vi "Open.vi"(6 "Start Counter":bool=TRUE, 7 "Allow multiple opens?":bool, 8 "error in (no error)":errorcluster, 9 "Encoder Signal Mode":T1, 10 "Channel Name":tag) -> (0 "error out":errorcluster, 3 "Encoder Ref Out":T2)   [LabVIEW 2021, in "Encoder.lvlib"]
doc: "Opens a reference to an encoder channel. You must open a reference before you use an encoder channel to read and decode signals from an encoder."
uses:
  <vilib>/myRIO/Instrument Drivers/Onboard IO/Encoder/Encoder.lvlib
  <vilib>/myRIO/Instrument Drivers/Onboard IO/Encoder/typedefs/Encoder Reference.ctl
  <vilib>/myRIO/Common/Instrument Driver Framework/Utilities/typedefs/myRIO Generic Hardware Reference.ctl
  <vilib>/myRIO/Common/Instrument Driver Framework/Utilities/typedefs/Hardware Version Enum.ctl
  <vilib>/myRIO/Common/Instrument Driver Framework/Utilities/typedefs/myRIO v1.0 Reference.ctl
  <vilib>/myRIO/Common/Instrument Driver Framework/Utilities/typedefs/Generic FPGA Reference.ctl
  <vilib>/myRIO/Common/Instrument Driver Framework/myRIO v1.0/Encoder/typedefs/Encoder Channels Enum.ctl
  <vilib>/myRIO/Common/Instrument Driver Framework/myRIO v1.0/Encoder/typedefs/Encoder Signal Mode.ctl
  <vilib>/myRIO/Common/Instrument Driver Framework/myRIO v1.0/Encoder/typedefs/Encoder Configuration v1.0.ctl
  <vilib>/myRIO/Common/Instrument Driver Framework/Utilities/vis/Validate Channels.vi
  <vilib>/myRIO/Common/Instrument Driver Framework/myRIO v1.0/Encoder/vis/myRIO v1.0 Reserve Encoder.vi
  <vilib>/myRIO/Common/Instrument Driver Framework/myRIO v1.0/Encoder/vis/myRIO v1.0 Unreserve Encoder.vi
  <vilib>/myRIO/Common/Instrument Driver Framework/roboRIO v1.0/Encoder/vis/roboRIO v1.0 Reserve Encoder.vi
  <vilib>/myRIO/Common/Instrument Driver Framework/ELVIS III v1.0/Encoder/vis/ELVIS III v1.0 Reserve Encoder.vi
  <vilib>/myRIO/Common/Instrument Driver Framework/myRIO v1.0/Encoder/vis/myRIO v1.0 Build MUX Configuration Encoder.vi
  <vilib>/myRIO/Common/Instrument Driver Framework/myRIO v1.0/Resource Manager/vis/myRIO v1.0 Reserve Channel List.vi
  <vilib>/myRIO/Common/Instrument Driver Framework/myRIO v1.0/Resource Manager/vis/myRIO v1.0 Unreserve Channel List.vi
  <vilib>/myRIO/Common/Instrument Driver Framework/roboRIO v1.0/Encoder/vis/roboRIO v1.0 Build MUX Configuration Encoder.vi
  <vilib>/myRIO/Common/Instrument Driver Framework/roboRIO v1.0/Resource Manager/vis/roboRIO v1.0 Reserve Channel List.vi
  <vilib>/myRIO/Common/Instrument Driver Framework/ELVIS III v1.0/Encoder/vis/ELVIS III v1.0 Build MUX Configuration Encoder.vi
  <vilib>/myRIO/Common/Instrument Driver Framework/myRIO v1.0/Resource Manager/vis/myRIO v1.0 Create Configuration List.vi
  <vilib>/myRIO/Common/Instrument Driver Framework/myRIO v1.0/Resource Manager/vis/myRIO v1.0 Reserve Channel.vi
  <vilib>/myRIO/Common/Instrument Driver Framework/myRIO v1.0/Resource Manager/vis/myRIO v1.0 Unreserve Channel.vi
  <vilib>/myRIO/Common/Instrument Driver Framework/roboRIO v1.0/Resource Manager/vis/roboRIO v1.0 Create Configuration List.vi
  <vilib>/myRIO/Common/Instrument Driver Framework/roboRIO v1.0/Resource Manager/vis/roboRIO v1.0 Reserve Channel.vi
  <vilib>/myRIO/Common/Instrument Driver Framework/roboRIO v1.0/Resource Manager/vis/roboRIO v1.0 Unreserve Channel.vi
  <vilib>/myRIO/Common/Instrument Driver Framework/ELVIS III v1.0/Resource Manager/vis/ELVIS III v1.0 Create Configuration List.vi
  <vilib>/myRIO/Common/Instrument Driver Framework/myRIO v1.0/Resource Manager/vis/myRIO v1.0 Build Mutex Name.vi
  <vilib>/myRIO/Common/Instrument Driver Framework/roboRIO v1.0/Resource Manager/vis/roboRIO v1.0 Build Mutex Name.vi
  <vilib>/Utility/VariantDataType/GetNumericInfo.vi
  <vilib>/myRIO/Common/Instrument Driver Framework/Utilities/vis/IO Manager.vi
  <vilib>/myRIO/Common/Instrument Driver Framework/Utilities/vis/Configuration Manager.vi
  <vilib>/myRIO/Common/Instrument Driver Framework/myRIO v1.0/Resource Manager/vis/myRIO v1.0 Configure IO.vi
  <vilib>/myRIO/Common/Instrument Driver Framework/myRIO v1.0/myRIO v1.0 Close.vi
  <vilib>/myRIO/Common/Instrument Driver Framework/myRIO v1.0/Encoder/vis/myRIO v1.0 Shutdown Encoder.vi
  <vilib>/myRIO/Common/Instrument Driver Framework/roboRIO v1.0/Resource Manager/vis/roboRIO v1.0 Configure IO.vi
  <vilib>/myRIO/Common/Instrument Driver Framework/ELVIS III v1.0/Resource Manager/vis/ELVIS III v1.0 Reserve Channel List.vi
  <vilib>/myRIO/Common/Instrument Driver Framework/ELVIS III v1.0/Resource Manager/vis/ELVIS III v1.0 Configure IO.vi
  <vilib>/userdefined/High Color/nirio_resource_hc.ctl
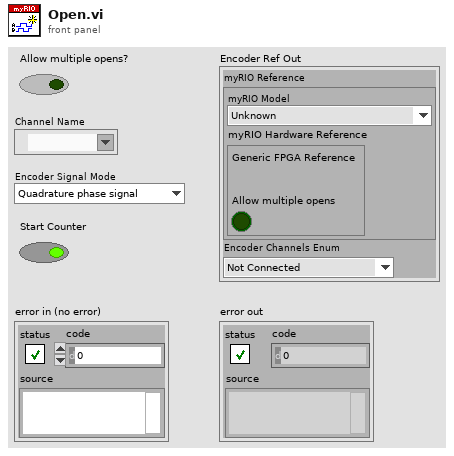
[diagram p1: front panel]
types:
  T1 = typedef "Encoder Signal Mode.ctl" = enum16{"Quadrature phase signal", "Step and direction signal"}
  T2 = typedef "Encoder.lvlib/Encoder Reference.ctl" = cluster{"myRIO Reference":T3, "Encoder Channels Enum":T7}
  T3 = typedef "myRIO Generic Hardware Reference.ctl" = cluster{"myRIO Model":T4, "myRIO Hardware Reference":T5}
  T4 = typedef "Hardware Version Enum.ctl" = enum16{"Unknown", "myRIO-1900", "myRIO-1950", "roboRIO", "NI ELVIS RIO CM", "ELVIS III"}
  T5 = typedef "myRIO v1.0 Reference.ctl" = cluster{"Generic FPGA Reference":T6, "Allow multiple opens":bool}
  T6 = typedef "Generic FPGA Reference.ctl" = refnum<k20>
  T7 = typedef "Encoder Channels Enum.ctl" = enum16{"Not Connected", "C/ENC0", "C/ENC1", "A/ENC", "A/ENC0", "A/ENC1", "A/ENC2", "A/ENC3", "A/ENC4", "A/ENC5", "A/ENC6", "A/ENC7", "A/ENC8", "A/ENC9", "B/ENC", "B/ENC0", "B/ENC1", "B/ENC2", "B/ENC3", "B/ENC4", "B/ENC5", "B/ENC6", "B/ENC7", "B/ENC8", "B/ENC9", "DIO/ENC0", "DIO/ENC1", "DIO/ENC2", "DIO/ENC3", "DIO/ENC4"}
  T8 = typedef "nirio_resource_hc.ctl" = tag
  T9 = typedef "Encoder Configuration v1.0.ctl" = cluster{"Encoder Signal Mode":T1, "Start Counter":bool}
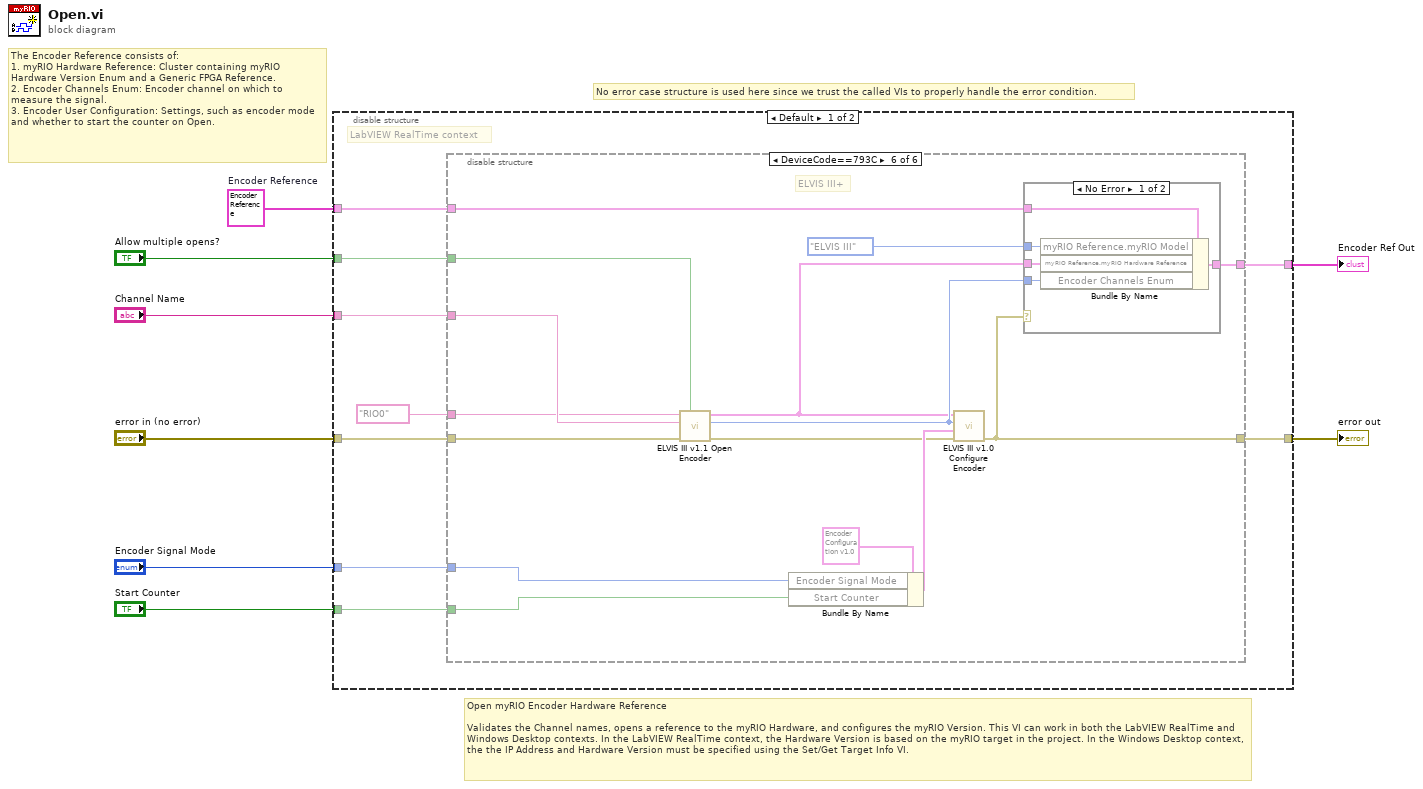
[diagram p0: block diagram]
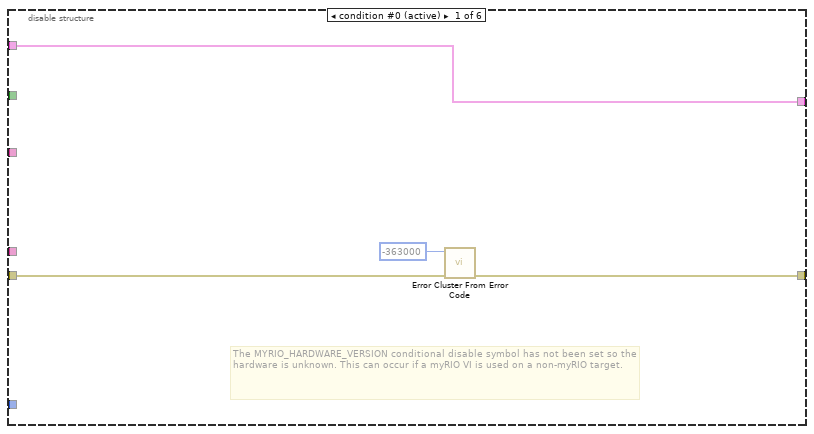
[diagram p2: hidden frame]
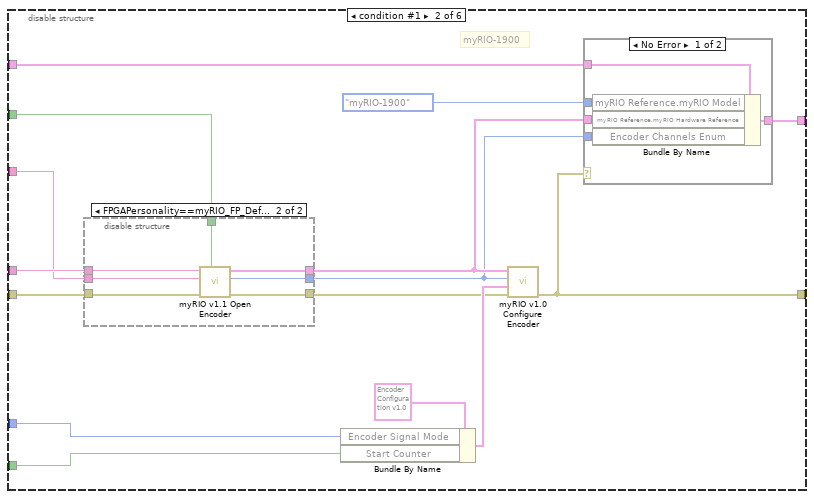
[diagram p3: hidden frame]
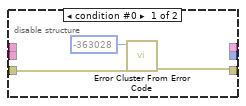
[diagram p4: hidden frame]
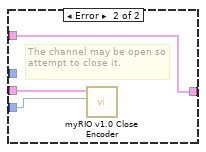
[diagram p5: hidden frame]
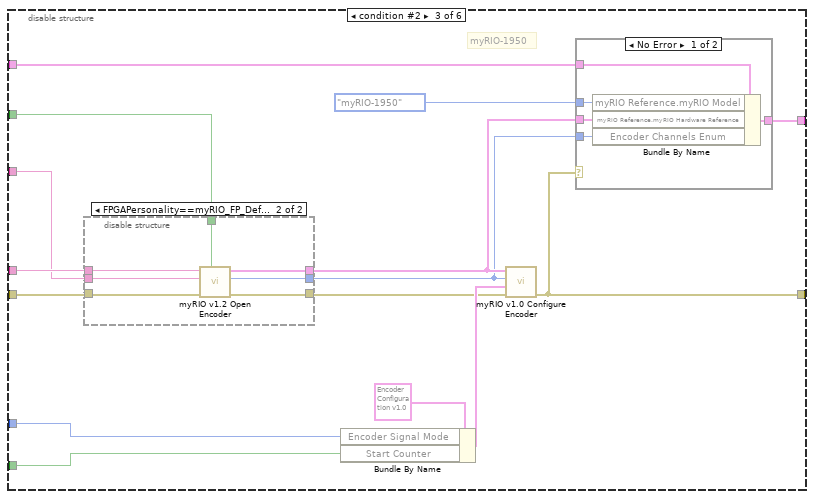
[diagram p6: hidden frame]
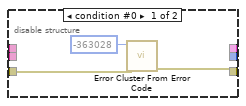
[diagram p7: hidden frame]
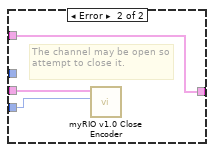
[diagram p8: hidden frame]
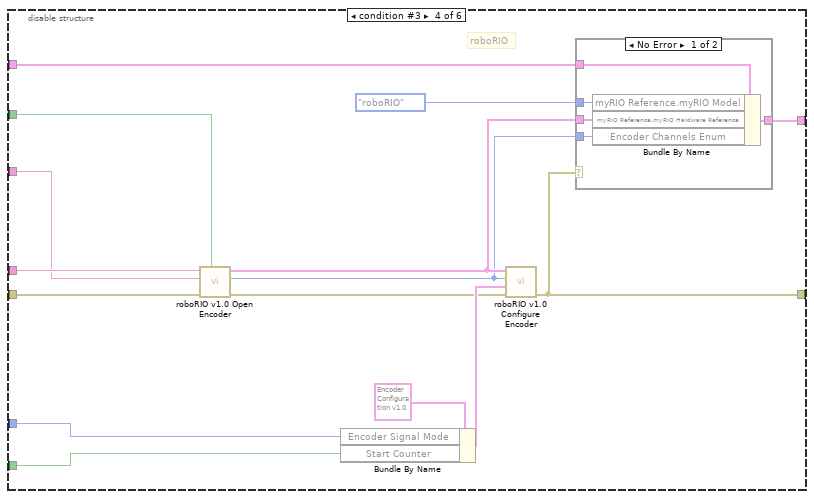
[diagram p9: hidden frame]
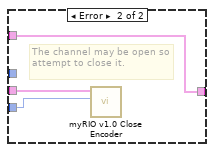
[diagram p10: hidden frame]
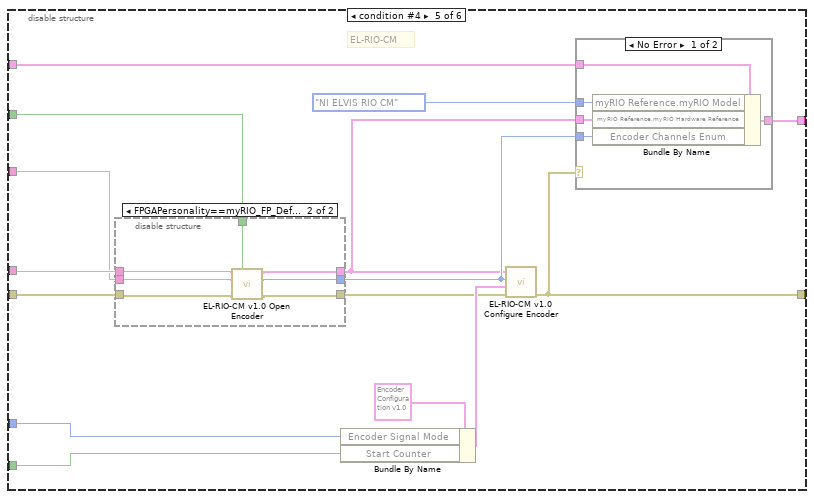
[diagram p11: hidden frame]
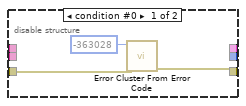
[diagram p12: hidden frame]
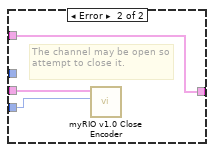
[diagram p13: hidden frame]
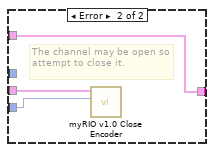
[diagram p14: hidden frame]
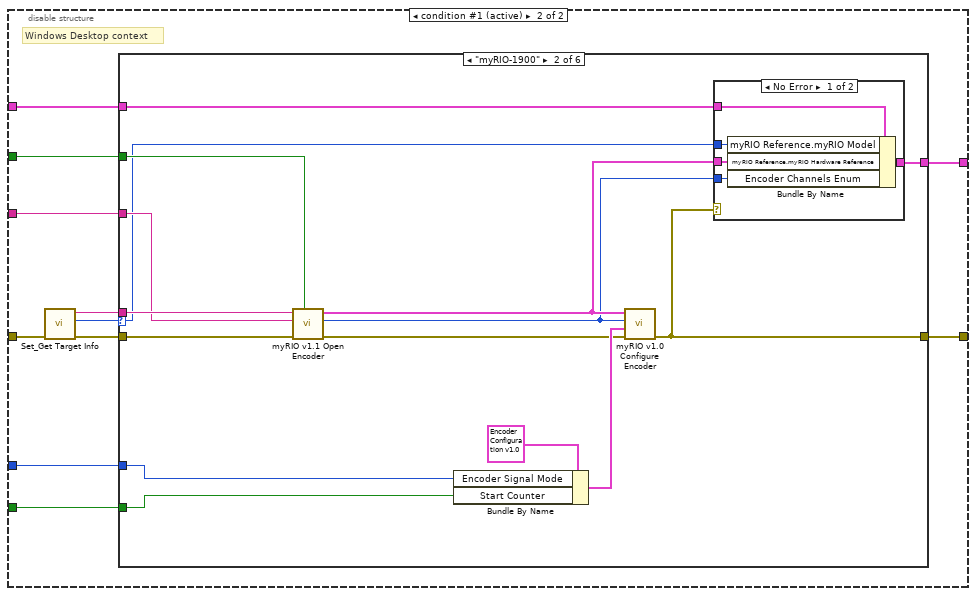
[diagram p15: hidden frame]
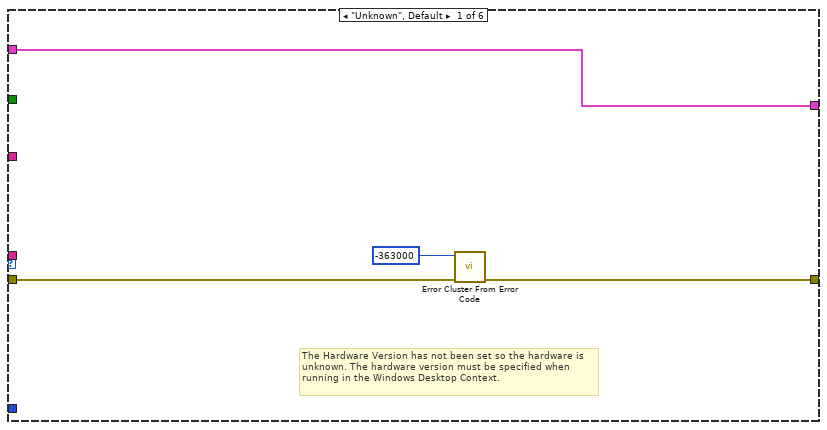
[diagram p16: hidden frame]
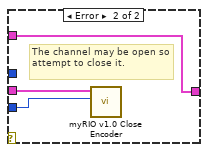
[diagram p17: hidden frame]
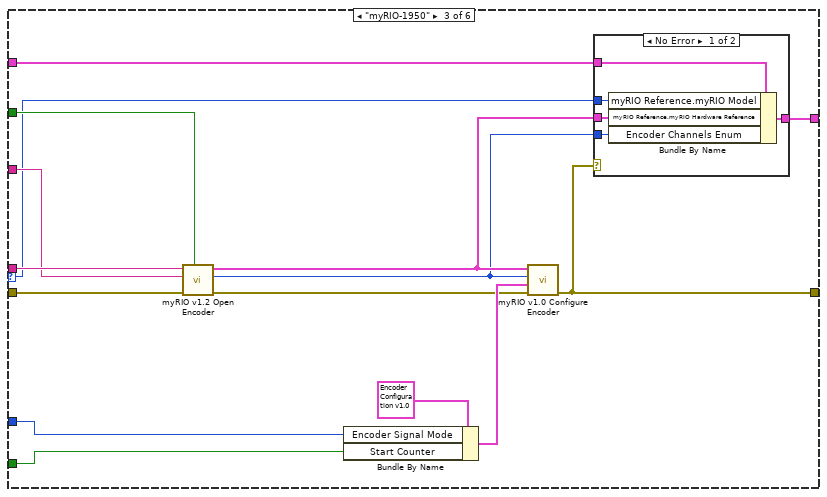
[diagram p18: hidden frame]
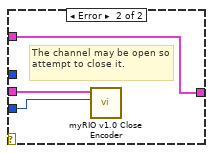
[diagram p19: hidden frame]
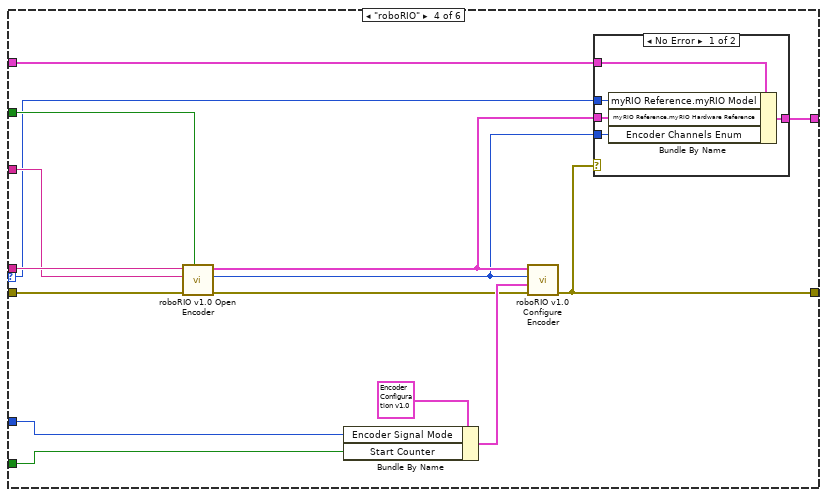
[diagram p20: hidden frame]
diagram:
  w8 = T2 {"myRIO Reference"={"myRIO Model"=enum."Unknown", "myRIO Hardware Reference"={"Generic FPGA Reference"=refnum, "Allow multiple opens"=FALSE}}, "Encoder Channels Enum"=enum."Not Connected"}  # Encoder Reference
  # "Open myRIO Encoder Hardware Reference\n\nValidates the Channel names, opens a reference to the myRIO Hardware, and configures the myRIO Version. This VI can work in both the LabVIEW RealTime and Windows Desktop contexts. In the LabVIEW RealTime context, the Hardware Version is based on the myRIO target in the project. In the Windows Desktop context, the the IP Address and Hardware Version must be specified using the Set/Get Target Info VI."
  # "No error case structure is used here since we trust the called VIs to properly handle the error condition."
  # "The Encoder Reference consists of:\n1. myRIO Hardware Reference: Cluster containing myRIO Hardware Version Enum and a Generic FPGA Reference.\n2. Encoder Channels Enum: Encoder channel on which to measure the signal.\n3. Encoder User Configuration: Settings, such as encoder mode and whether to start the counter on Open."
  n1 = disable-structure shown="Default" {
    disable-tunnel: [w17 w177] -> w6
    disable-tunnel: "error in (no error)" -> [w15 w172]
    disable-tunnel: [w14 w176] -> w5
    disable-tunnel: w8 -> [w12 w175]
    disable-tunnel: "Encoder Signal Mode" -> [w13 w174]
    disable-tunnel: "Start Counter" -> [w11 w173]
    disable-tunnel: "Channel Name" -> [w9 w167]
    disable-tunnel: "Allow multiple opens?" -> [w10 w168]
    frame condition #0 {
      # "LabVIEW RealTime context"
      n2 = disable-structure shown="DeviceCode==793C" {
        disable-tunnel: [w20 w22 w55 w88 w118 w145] -> w17
        disable-tunnel: [w18 w31 w64 w97 w123 w144] -> w14
        disable-tunnel: T8 "RIO0" ("resource name") -> [_ w33 w66 w99 w114 w149]
        disable-tunnel: w15 -> [w19 w32 w65 w98 w112 w148]
        disable-tunnel: w13 -> [_ w29 w62 w95 w121 w147]
        disable-tunnel: w12 -> [w18 w27 w60 w93 w119 w152]
        disable-tunnel: w11 -> [_ w28 w61 w94 w120 w146]
        disable-tunnel: w10 -> [_ w23 w56 w89 w111 w151]
        disable-tunnel: w9 -> [_ w25 w58 w91 w113 w150]
        frame condition #0 (active) {
          # "The MYRIO_HARDWARE_VERSION conditional disable symbol has not been set so the hardware is unknown. This can occur if a myRIO VI is used on a non-myRIO target."
          n3 = call <vilib>:"Error Cluster From Error Code.vi"("error in (no error)"=w19, "error code (0)"=-363000) -> ("error out"=w20:errorcluster)  [unwired: 7 in]
        }
        frame condition #1 {
          # "myRIO-1900"
          n4 = disable-structure shown="FPGAPersonality==myRIO_FP_Default, Default" {
            disable-tunnel: [_ w46] -> w35
            disable-tunnel: w33 -> [_ w45]
            disable-tunnel: w32 -> [w38 w44]
            disable-tunnel: [w37 w43] -> w26
            disable-tunnel: w25 -> [_ w42]
            disable-tunnel: [_ w41] -> w24
            disable-tunnel: w23 -> [_ w40]
            frame condition #0 {
              n5 = call <vilib>:"Error Cluster From Error Code.vi"("error in (no error)"=w38, "error code (0)"=-363028) -> ("error out"=w37:errorcluster)  [unwired: 7 in]
            }
            frame condition #1 (active) {
              n6 = call <vilib>:"myRIO v1.1 Open Encoder.vi"("Allow multiple opens?"=w40, "error in (no error)"=w44, "Channel Name"=w42, "Resource name"=w45) -> ("error out"=w43:errorcluster, "Encoder Channel"=w41:T7, "myRIO Ref Out"=w46:T5)  [unwired: 5 in]
            }
          }
          n7 = Bundle By Name(cluster=T9 {"Encoder Signal Mode"=enum."Quadrature phase signal", "Start Counter"=FALSE} ("PWM Configuration"), "Encoder Signal Mode"=w29, "Start Counter"=w28) -> (w30:T9)
          n8 = call <vilib>:"myRIO v1.0 Configure Encoder.vi"("error in (no error)"=w26, "Encoder Configuration v1.0"=w30, "Encoder Channel"=w24, "myRIO Ref In"=w35) -> ("error out"=w22:errorcluster)  [unwired: 7 in]
          n9 = case shown="No Error" w22 {
            tunnel: Hardware_Version_Enum."myRIO-1900" ("Hardware Version") -> [w51 _]
            tunnel: w35 -> [w50 w53]
            tunnel: [w49 w54] -> w31
            tunnel: w27 -> [w48 w54]
            tunnel: w24 -> [w47 w52]
            frame No Error {
              n10 = Bundle By Name(cluster=w48, "myRIO Reference.myRIO Model"=w51, "myRIO Reference.myRIO Hardware Reference"=w50, "Encoder Channels Enum"=w47) -> (w49:T2)
            }
            frame Error {
              # "The channel may be open so attempt to close it."
              n11 = call <vilib>:"myRIO v1.0 Close Encoder.vi"("Encoder Channel"=w52, "myRIO Ref In"=w53) -> ()  [unwired: 9 in, 1 out]
            }
          }
        }
        frame condition #2 {
          # "myRIO-1950"
          n12 = disable-structure shown="FPGAPersonality==myRIO_FP_Default, Default" {
            disable-tunnel: [_ w79] -> w68
            disable-tunnel: w66 -> [_ w78]
            disable-tunnel: w65 -> [w71 w77]
            disable-tunnel: [w70 w76] -> w59
            disable-tunnel: w58 -> [_ w75]
            disable-tunnel: [_ w74] -> w57
            disable-tunnel: w56 -> [_ w73]
            frame condition #0 {
              n13 = call <vilib>:"Error Cluster From Error Code.vi"("error in (no error)"=w71, "error code (0)"=-363028) -> ("error out"=w70:errorcluster)  [unwired: 7 in]
            }
            frame condition #1 (active) {
              n14 = call <vilib>:"myRIO v1.2 Open Encoder.vi"("Allow multiple opens?"=w73, "error in (no error)"=w77, "Channel Name"=w75, "Resource name"=w78) -> ("error out"=w76:errorcluster, "Encoder Channel"=w74:T7, "myRIO Ref Out"=w79:T5)  [unwired: 5 in]
            }
          }
          n15 = Bundle By Name(cluster=T9 {"Encoder Signal Mode"=enum."Quadrature phase signal", "Start Counter"=FALSE} ("PWM Configuration"), "Encoder Signal Mode"=w62, "Start Counter"=w61) -> (w63:T9)
          n16 = call <vilib>:"myRIO v1.0 Configure Encoder.vi"("error in (no error)"=w59, "Encoder Configuration v1.0"=w63, "Encoder Channel"=w57, "myRIO Ref In"=w68) -> ("error out"=w55:errorcluster)  [unwired: 7 in]
          n17 = case shown="No Error" w55 {
            tunnel: Hardware_Version_Enum."myRIO-1950" ("Hardware Version") -> [w84 _]
            tunnel: w68 -> [w83 w86]
            tunnel: [w82 w87] -> w64
            tunnel: w60 -> [w81 w87]
            tunnel: w57 -> [w80 w85]
            frame No Error {
              n18 = Bundle By Name(cluster=w81, "myRIO Reference.myRIO Model"=w84, "myRIO Reference.myRIO Hardware Reference"=w83, "Encoder Channels Enum"=w80) -> (w82:T2)
            }
            frame Error {
              # "The channel may be open so attempt to close it."
              n19 = call <vilib>:"myRIO v1.0 Close Encoder.vi"("Encoder Channel"=w85, "myRIO Ref In"=w86) -> ()  [unwired: 9 in, 1 out]
            }
          }
        }
        frame condition #3 {
          # "roboRIO"
          n20 = call <vilib>:"roboRIO v1.0 Open Encoder.vi"("Allow multiple opens?"=w89, "error in (no error)"=w98, "Channel Name"=w91, "Resource name"=w99) -> ("error out"=w92:errorcluster, "Encoder Channel"=w90:T7, "myRIO Ref Out"=w101:T5)  [unwired: 5 in]
          n21 = Bundle By Name(cluster=T9 {"Encoder Signal Mode"=enum."Quadrature phase signal", "Start Counter"=FALSE} ("PWM Configuration"), "Encoder Signal Mode"=w95, "Start Counter"=w94) -> (w96:T9)
          n22 = call <vilib>:"roboRIO v1.0 Configure Encoder.vi"("error in (no error)"=w92, "Encoder Configuration v1.0"=w96, "Encoder Channel"=w90, "myRIO Ref In"=w101) -> ("error out"=w88:errorcluster)  [unwired: 7 in]
          n23 = case shown="No Error" w88 {
            tunnel: Hardware_Version_Enum."roboRIO" ("Hardware Version") -> [w107 _]
            tunnel: w101 -> [w106 w109]
            tunnel: [w105 w110] -> w97
            tunnel: w93 -> [w104 w110]
            tunnel: w90 -> [w103 w108]
            frame No Error {
              n24 = Bundle By Name(cluster=w104, "myRIO Reference.myRIO Model"=w107, "myRIO Reference.myRIO Hardware Reference"=w106, "Encoder Channels Enum"=w103) -> (w105:T2)
            }
            frame Error {
              # "The channel may be open so attempt to close it."
              n25 = call <vilib>:"myRIO v1.0 Close Encoder.vi"("Encoder Channel"=w108, "myRIO Ref In"=w109) -> ()  [unwired: 9 in, 1 out]
            }
          }
        }
        frame condition #4 {
          # "EL-RIO-CM"
          n26 = disable-structure shown="FPGAPersonality==myRIO_FP_Default, Default" {
            disable-tunnel: [_ w133] -> w115
            disable-tunnel: w114 -> [_ w131]
            disable-tunnel: w112 -> [w127 w129]
            disable-tunnel: [w126 w135] -> w117
            disable-tunnel: w113 -> [_ w130]
            disable-tunnel: [_ w134] -> w116
            disable-tunnel: w111 -> [_ w132]
            frame condition #0 {
              n27 = call <vilib>:"Error Cluster From Error Code.vi"("error in (no error)"=w127, "error code (0)"=-363028) -> ("error out"=w126:errorcluster)  [unwired: 7 in]
            }
            frame condition #1 (active) {
              n28 = call <vilib>:"EL-RIO-CM v1.0 Open Encoder.vi"("Allow multiple opens?"=w132, "error in (no error)"=w129, "Channel Name"=w130, "Resource name"=w131) -> ("error out"=w135:errorcluster, "Encoder Channel"=w134:T7, "myRIO Ref Out"=w133:T5)  [unwired: 5 in]
            }
          }
          n29 = Bundle By Name(cluster=T9 {"Encoder Signal Mode"=enum."Quadrature phase signal", "Start Counter"=FALSE} ("PWM Configuration"), "Encoder Signal Mode"=w121, "Start Counter"=w120) -> (w122:T9)
          n30 = call <vilib>:"EL-RIO-CM v1.0 Configure Encoder.vi"("error in (no error)"=w117, "Encoder Configuration v1.0"=w122, "Encoder Channel"=w116, "myRIO Ref In"=w115) -> ("error out"=w118:errorcluster)  [unwired: 7 in]
          n31 = case shown="No Error" w118 {
            tunnel: Hardware_Version_Enum."NI ELVIS RIO CM" ("Hardware Version") -> [w140 _]
            tunnel: w115 -> [w139 w142]
            tunnel: [w138 w143] -> w123
            tunnel: w119 -> [w137 w143]
            tunnel: w116 -> [w136 w141]
            frame No Error {
              n32 = Bundle By Name(cluster=w137, "myRIO Reference.myRIO Model"=w140, "myRIO Reference.myRIO Hardware Reference"=w139, "Encoder Channels Enum"=w136) -> (w138:T2)
            }
            frame Error {
              # "The channel may be open so attempt to close it."
              n33 = call <vilib>:"myRIO v1.0 Close Encoder.vi"("Encoder Channel"=w141, "myRIO Ref In"=w142) -> ()  [unwired: 9 in, 1 out]
            }
          }
        }
        frame condition #5 {
          # "ELVIS III+"
          n34 = call <vilib>:"ELVIS III v1.1 Open Encoder.vi"("Allow multiple opens?"=w151, "error in (no error)"=w148, "Channel Name"=w150, "Resource name"=w149) -> ("error out"=w155:errorcluster, "Encoder Channel"=w154:T7, "myRIO Ref Out"=w153:T5)  [unwired: 5 in]
          n35 = Bundle By Name(cluster=T9 {"Encoder Signal Mode"=enum."Quadrature phase signal", "Start Counter"=FALSE} ("PWM Configuration"), "Encoder Signal Mode"=w147, "Start Counter"=w146) -> (w156:T9)
          n36 = call <vilib>:"ELVIS III v1.0 Configure Encoder.vi"("error in (no error)"=w155, "Encoder Configuration v1.0"=w156, "Encoder Channel"=w154, "myRIO Ref In"=w153) -> ("error out"=w145:errorcluster)  [unwired: 7 in]
          n37 = case shown="No Error" w145 {
            tunnel: Hardware_Version_Enum."ELVIS III" ("Hardware Version") -> [w163 _]
            tunnel: w153 -> [w162 w165]
            tunnel: [w161 w166] -> w144
            tunnel: w152 -> [w160 w166]
            tunnel: w154 -> [w159 w164]
            frame No Error {
              n38 = Bundle By Name(cluster=w160, "myRIO Reference.myRIO Model"=w163, "myRIO Reference.myRIO Hardware Reference"=w162, "Encoder Channels Enum"=w159) -> (w161:T2)
            }
            frame Error {
              # "The channel may be open so attempt to close it."
              n39 = call <vilib>:"myRIO v1.0 Close Encoder.vi"("Encoder Channel"=w164, "myRIO Ref In"=w165) -> ()  [unwired: 9 in, 1 out]
            }
          }
        }
      }
    }
    frame condition #1 (active) {
      # "Windows Desktop context"
      n40 = call <vilib>:"Set_Get Target Info.vi"("error in (no error)"=w172) -> ("error out"=w171:errorcluster, "Hardware Version"=w169:T4, "IP Address"=w170:string)  [unwired: 8 in]
      n41 = case shown="\"myRIO-1900\"" w169 {
        selector: w169 -> [_ w182 w205 w228 w251 w279]
        tunnel: [w180 w183 w206 w229 w252 w275] -> w177
        tunnel: w170 -> [_ w195 w218 w241 w264 w280]
        tunnel: w171 -> [w179 w194 w217 w240 w263 w278]
        tunnel: [w178 w193 w216 w239 w262 w274] -> w176
        tunnel: w175 -> [w178 w190 w213 w236 w259 w283]
        tunnel: w174 -> [_ w188 w211 w234 w257 w277]
        tunnel: w173 -> [_ w189 w212 w235 w258 w276]
        tunnel: w168 -> [_ w184 w207 w230 w253 w282]
        tunnel: w167 -> [_ w186 w209 w232 w255 w281]
        frame "Unknown", Default {
          # "The Hardware Version has not been set so the hardware is unknown. The hardware version must be specified when running in the Windows Desktop Context."
          n42 = call <vilib>:"Error Cluster From Error Code.vi"("error in (no error)"=w179, "error code (0)"=-363000) -> ("error out"=w180:errorcluster)  [unwired: 7 in]
        }
        frame "myRIO-1900" {
          n43 = call <vilib>:"myRIO v1.1 Open Encoder.vi"("Allow multiple opens?"=w184, "error in (no error)"=w194, "Channel Name"=w186, "Resource name"=w195) -> ("error out"=w187:errorcluster, "Encoder Channel"=w185:T7, "myRIO Ref Out"=w196:T5)  [unwired: 5 in]
          n44 = Bundle By Name(cluster=T9 {"Encoder Signal Mode"=enum."Quadrature phase signal", "Start Counter"=FALSE} ("PWM Configuration"), "Encoder Signal Mode"=w188, "Start Counter"=w189) -> (w191:T9)
          n45 = call <vilib>:"myRIO v1.0 Configure Encoder.vi"("error in (no error)"=w187, "Encoder Configuration v1.0"=w191, "Encoder Channel"=w185, "myRIO Ref In"=w196) -> ("error out"=w183:errorcluster)  [unwired: 7 in]
          n46 = case shown="No Error" w183 {
            tunnel: w182 -> [w201 _]
            tunnel: w196 -> [w200 w203]
            tunnel: [w199 w204] -> w193
            tunnel: w190 -> [w198 w204]
            tunnel: w185 -> [w197 w202]
            frame No Error {
              n47 = Bundle By Name(cluster=w198, "myRIO Reference.myRIO Model"=w201, "myRIO Reference.myRIO Hardware Reference"=w200, "Encoder Channels Enum"=w197) -> (w199:T2)
            }
            frame Error {
              # "The channel may be open so attempt to close it."
              n48 = call <vilib>:"myRIO v1.0 Close Encoder.vi"("Encoder Channel"=w202, "myRIO Ref In"=w203) -> ()  [unwired: 9 in, 1 out]
            }
          }
        }
        frame "myRIO-1950" {
          n49 = call <vilib>:"myRIO v1.2 Open Encoder.vi"("Allow multiple opens?"=w207, "error in (no error)"=w217, "Channel Name"=w209, "Resource name"=w218) -> ("error out"=w210:errorcluster, "Encoder Channel"=w208:T7, "myRIO Ref Out"=w219:T5)  [unwired: 5 in]
          n50 = Bundle By Name(cluster=T9 {"Encoder Signal Mode"=enum."Quadrature phase signal", "Start Counter"=FALSE} ("PWM Configuration"), "Encoder Signal Mode"=w211, "Start Counter"=w212) -> (w214:T9)
          n51 = call <vilib>:"myRIO v1.0 Configure Encoder.vi"("error in (no error)"=w210, "Encoder Configuration v1.0"=w214, "Encoder Channel"=w208, "myRIO Ref In"=w219) -> ("error out"=w206:errorcluster)  [unwired: 7 in]
          n52 = case shown="No Error" w206 {
            tunnel: w205 -> [w224 _]
            tunnel: w219 -> [w223 w226]
            tunnel: [w222 w227] -> w216
            tunnel: w213 -> [w221 w227]
            tunnel: w208 -> [w220 w225]
            frame No Error {
              n53 = Bundle By Name(cluster=w221, "myRIO Reference.myRIO Model"=w224, "myRIO Reference.myRIO Hardware Reference"=w223, "Encoder Channels Enum"=w220) -> (w222:T2)
            }
            frame Error {
              # "The channel may be open so attempt to close it."
              n54 = call <vilib>:"myRIO v1.0 Close Encoder.vi"("Encoder Channel"=w225, "myRIO Ref In"=w226) -> ()  [unwired: 9 in, 1 out]
            }
          }
        }
        frame "roboRIO" {
          n55 = call <vilib>:"roboRIO v1.0 Open Encoder.vi"("Allow multiple opens?"=w230, "error in (no error)"=w240, "Channel Name"=w232, "Resource name"=w241) -> ("error out"=w233:errorcluster, "Encoder Channel"=w231:T7, "myRIO Ref Out"=w242:T5)  [unwired: 5 in]
          n56 = Bundle By Name(cluster=T9 {"Encoder Signal Mode"=enum."Quadrature phase signal", "Start Counter"=FALSE} ("PWM Configuration"), "Encoder Signal Mode"=w234, "Start Counter"=w235) -> (w237:T9)
          n57 = call <vilib>:"roboRIO v1.0 Configure Encoder.vi"("error in (no error)"=w233, "Encoder Configuration v1.0"=w237, "Encoder Channel"=w231, "myRIO Ref In"=w242) -> ("error out"=w229:errorcluster)  [unwired: 7 in]
          n58 = case shown="No Error" w229 {
            tunnel: w228 -> [w247 _]
            tunnel: w242 -> [w246 w249]
            tunnel: [w245 w250] -> w239
            tunnel: w236 -> [w244 w250]
            tunnel: w231 -> [w243 w248]
            frame No Error {
              n59 = Bundle By Name(cluster=w244, "myRIO Reference.myRIO Model"=w247, "myRIO Reference.myRIO Hardware Reference"=w246, "Encoder Channels Enum"=w243) -> (w245:T2)
            }
            frame Error {
              # "The channel may be open so attempt to close it."
              n60 = call <vilib>:"myRIO v1.0 Close Encoder.vi"("Encoder Channel"=w248, "myRIO Ref In"=w249) -> ()  [unwired: 9 in, 1 out]
            }
          }
        }
        frame "NI ELVIS RIO CM" {
          n61 = call <vilib>:"EL-RIO-CM v1.0 Open Encoder.vi"("Allow multiple opens?"=w253, "error in (no error)"=w263, "Channel Name"=w255, "Resource name"=w264) -> ("error out"=w256:errorcluster, "Encoder Channel"=w254:T7, "myRIO Ref Out"=w265:T5)  [unwired: 5 in]
          n62 = Bundle By Name(cluster=T9 {"Encoder Signal Mode"=enum."Quadrature phase signal", "Start Counter"=FALSE} ("PWM Configuration"), "Encoder Signal Mode"=w257, "Start Counter"=w258) -> (w260:T9)
          n63 = call <vilib>:"EL-RIO-CM v1.0 Configure Encoder.vi"("error in (no error)"=w256, "Encoder Configuration v1.0"=w260, "Encoder Channel"=w254, "myRIO Ref In"=w265) -> ("error out"=w252:errorcluster)  [unwired: 7 in]
          n64 = case shown="No Error" w252 {
            tunnel: w251 -> [w270 _]
            tunnel: w265 -> [w269 w272]
            tunnel: [w268 w273] -> w262
            tunnel: w259 -> [w267 w273]
            tunnel: w254 -> [w266 w271]
            frame No Error {
              n65 = Bundle By Name(cluster=w267, "myRIO Reference.myRIO Model"=w270, "myRIO Reference.myRIO Hardware Reference"=w269, "Encoder Channels Enum"=w266) -> (w268:T2)
            }
            frame Error {
              # "The channel may be open so attempt to close it."
              n66 = call <vilib>:"myRIO v1.0 Close Encoder.vi"("Encoder Channel"=w271, "myRIO Ref In"=w272) -> ()  [unwired: 9 in, 1 out]
            }
          }
        }
        frame "ELVIS III" {
          n67 = call <vilib>:"ELVIS III v1.1 Open Encoder.vi"("Allow multiple opens?"=w282, "error in (no error)"=w278, "Channel Name"=w281, "Resource name"=w280) -> ("error out"=w285:errorcluster, "Encoder Channel"=w284:T7, "myRIO Ref Out"=w288:T5)  [unwired: 5 in]
          n68 = Bundle By Name(cluster=T9 {"Encoder Signal Mode"=enum."Quadrature phase signal", "Start Counter"=FALSE} ("PWM Configuration"), "Encoder Signal Mode"=w277, "Start Counter"=w276) -> (w286:T9)
          n69 = call <vilib>:"ELVIS III v1.0 Configure Encoder.vi"("error in (no error)"=w285, "Encoder Configuration v1.0"=w286, "Encoder Channel"=w284, "myRIO Ref In"=w288) -> ("error out"=w275:errorcluster)  [unwired: 7 in]
          n70 = case shown="No Error" w275 {
            tunnel: w279 -> [w293 _]
            tunnel: w288 -> [w292 w295]
            tunnel: [w291 w296] -> w274
            tunnel: w283 -> [w290 w296]
            tunnel: w284 -> [w289 w294]
            frame No Error {
              n71 = Bundle By Name(cluster=w290, "myRIO Reference.myRIO Model"=w293, "myRIO Reference.myRIO Hardware Reference"=w292, "Encoder Channels Enum"=w289) -> (w291:T2)
            }
            frame Error {
              # "The channel may be open so attempt to close it."
              n72 = call <vilib>:"myRIO v1.0 Close Encoder.vi"("Encoder Channel"=w294, "myRIO Ref In"=w295) -> ()  [unwired: 9 in, 1 out]
            }
          }
        }
      }
    }
  }
  "Encoder Ref Out" <- w5
  "error out" <- w6
